vi "ex_SecondsToHMS.vi"(0 "seconds":i32) -> (1 "hours":i32, 2 "minutes":i32, 3 "seconds":i32)   [LabVIEW 2020]
doc: "Converts a decimal value representing seconds to the appropriate number of hours, minutes, and seconds."
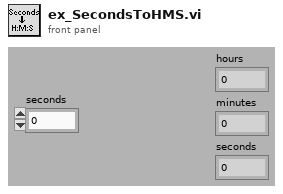
[diagram p1: front panel]
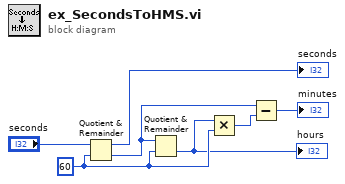
[diagram p0: block diagram]
diagram:
  w4 = 60 ("seconds")
  n1 = Quotient & Remainder(x="seconds", y=w4) -> (x-y*floor(x/y)=→"seconds":i32, floor(x/y)=w5:i32)
  n2 = Quotient & Remainder(x=w5, y=w4) -> (floor(x/y)=w3:i32)  [unwired: 1 out]
  "hours" <- w3
  n3 = Multiply(x=w3, y=w4) -> (x*y=w1:i32)
  n4 = Subtract(x=w5, y=w1) -> (x-y=→"minutes":i32)
